vi "raptor_initialise.vi"(8 "error in (no error)":errorcluster, 10 "Buffer Size":i32=40, 11 "Raptor Parameters":T1={"Vertical Search Range"=0, "Template Width"=0, "Template Height"=0, "Correlation Threshold"=0.0, "Surface Morph Size"=0, "En Face Width"=0, "En Face Height"=0, "En Face Depth"=0, "Aspect Ratio"=0.0, "Continous Scan"=FALSE, "Num En Face Reviews"=0, "Fluoresence Channel"=FALSE, "Track Depth"=FALSE, "Auto Expand"=FALSE, "Show Raptor Window"=TRUE, "Surface Threshold"=0, "Gaussian Filter Size"=0.0, "Mean Filter Size"=0.0}) -> (0 "error out":errorcluster)   [LabVIEW 2016]
doc: "Raptor: Call to begin using Raptor. Pass a full set of Raptor parameters."
uses:
  typedef/raptor_parameters.ctl
  typedef/raptor_image.ctl
  <vilib>/vision/Image Controls.llb/IMAQ Image.ctl
  globals/Channel 1 Image Ring.vi
  globals/Channel 2 Image Ring.vi
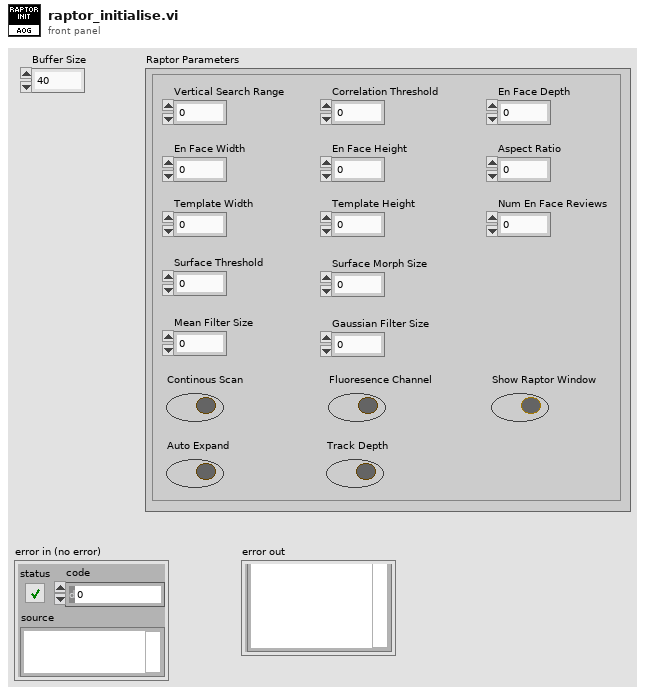
[diagram p1: front panel]
types:
  T1 = typedef "raptor_parameters.ctl" = cluster{"Vertical Search Range":i32, "Template Width":i32, "Template Height":i32, "Correlation Threshold":dbl, "Surface Morph Size":i32, "En Face Width":i32, "En Face Height":i32, "En Face Depth":i32, "Aspect Ratio":dbl, "Continous Scan":bool, "Num En Face Reviews":i32, "Fluoresence Channel":bool, "Track Depth":bool, "Auto Expand":bool, "Show Raptor Window":bool, "Surface Threshold":i32, "Gaussian Filter Size":dbl, "Mean Filter Size":dbl}
  T2 = typedef "raptor_image.ctl" = cluster{"Data":variant, "Image":T3}
  T3 = typedef "IMAQ Image.ctl" = refnum<image>
  T4 = typedef "Image Type" = u32
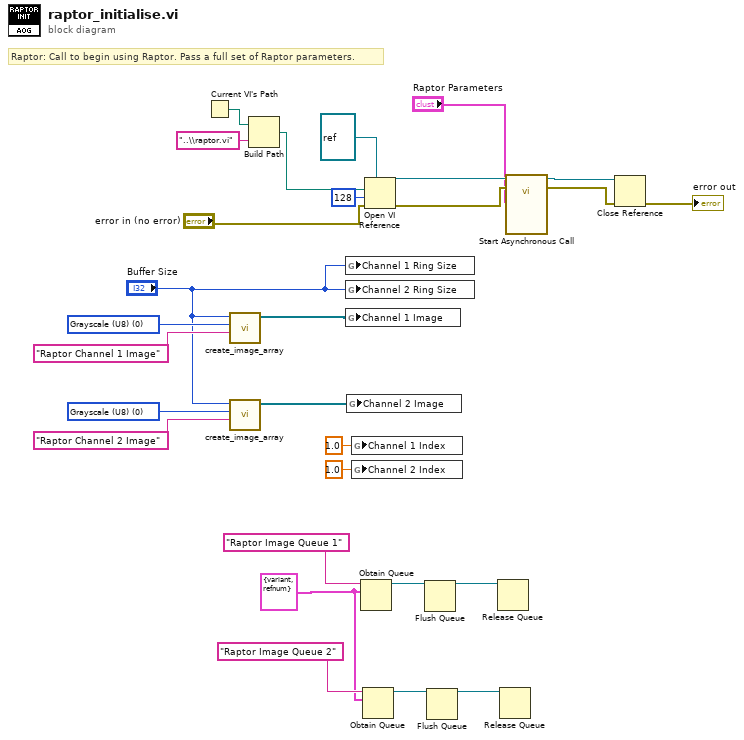
[diagram p0: block diagram]
diagram:
  w2 = T2 {"Data"=variant, "Image"=refnum} ("Cluster")
  w16 = T4 0 items=["Grayscale (U8)", "Grayscale (I16)", "Grayscale (SGL)", "Complex (CSG)", "RGB (U32)", "HSL (U32)", "RGB (U64)", "Grayscale (U16)"] ("Image Type")
  w19 = T4 0 items=["Grayscale (U8)", "Grayscale (I16)", "Grayscale (SGL)", "Complex (CSG)", "RGB (U32)", "HSL (U32)", "RGB (U64)", "Grayscale (U16)"] ("Image Type")
  # "Raptor: Call to begin using Raptor. Pass a full set of Raptor parameters."
  n1 = Current VI's Path() -> (path=w23:path)
  n2 = call "create_image_array.vi"("Prefix"="Raptor Channel 1 Image", "Image Type"=w19, "Num Images"="Buffer Size") -> ("Image Array"=w15:T3[])  [unwired: 7 in, 1 out]
  n3 = call "create_image_array.vi"("Prefix"="Raptor Channel 2 Image", "Image Type"=w16, "Num Images"="Buffer Size") -> ("Image Array"=w14:T3[])  [unwired: 7 in, 1 out]
  n4 = Build Path(base path=w23, name or relative path="..\\raptor.vi") -> (appended path=w21:path)
  n5 = global write "Channel 1 Image Ring.vi" "Channel 1 Ring Size"("Buffer Size") -> ()
  n6 = global write "Channel 2 Image Ring.vi" "Channel 2 Ring Size"("Buffer Size") -> ()
  n7 = global write "Channel 1 Image Ring.vi" "Channel 1 Image"(w15) -> ()
  n8 = global write "Channel 2 Image Ring.vi" "Channel 2 Image"(w14) -> ()
  n9 = global write "Channel 1 Image Ring.vi" "Channel 1 Index"(1.0 ("Channel 1 Index")) -> ()
  n10 = global write "Channel 2 Image Ring.vi" "Channel 2 Index"(1.0 ("Channel 2 Index")) -> ()
  n11 = Obtain Queue(name (unnamed)="Raptor Image Queue 1", element data type=w2) -> (queue out=w7:refnum<queue>)  [unwired: 3 in, 2 out]
  n12 = Obtain Queue(name (unnamed)="Raptor Image Queue 2", element data type=w2) -> (queue out=w4:refnum<queue>)  [unwired: 3 in, 2 out]
  n13 = Open VI Reference(type specifier VI Refnum (for type only)=refnum<vi> refnum, vi path=w21, options=128, error in (no error)="error in (no error)") -> (vi reference=w28:refnum<vi>, error out=w27:errorcluster)  [unwired: 2 in]
  n14 = Flush Queue(queue=w7) -> (queue out=w6:refnum<queue>)  [unwired: 1 in, 2 out]
  n15 = Flush Queue(queue=w4) -> (queue out=w5:refnum<queue>)  [unwired: 1 in, 2 out]
  n16 = Release Queue(queue=w6) -> ()  [unwired: 2 in, 3 out]
  n17 = Release Queue(queue=w5) -> ()  [unwired: 2 in, 3 out]
  n18 = call-by-ref "Start Asynchronous Call"(reference=w28, error in=w27, "Raptor Parameters"="Raptor Parameters") -> (reference out=w26:refnum<vi>, error out=w25:errorcluster)  [unwired: 11 in]
  n19 = Close Reference(reference=w26, error in (no error)=w25) -> (error out=→"error out":errorcluster)
